vi "Calculate IV Average.vi"(8 "error in (no error)":errorcluster, 9 "Time Offset, s (0)":dbl format="%#_6p", 10 "Supply Line Handle in":refnum<k15>, 11 "Supply Line Measurements Results in":T1 {"Power (W)" format="%#_6p"; "Current (A)" format="%#_6p"; "Voltage (V)" format="%#_6p"}) -> (0 "error out":errorcluster, 3 "Supply Line Measurements Results out":T1 {"Power (W)" format="%#_6p"; "Current (A)" format="%#_6p"; "Voltage (V)" format="%#_6p"})   [LabVIEW 2016, in "RDLUtilities.lvlib"]
uses:
  RDLUtilities.lvlib
  Supply/Typedefs/Measurement Results.ctl
  <vilib>/Analysis/baseanly.llb/Mean (DBL).vi
  <vilib>/Analysis/NI_AALBase.lvlib
  Supply/Supply.lvlib
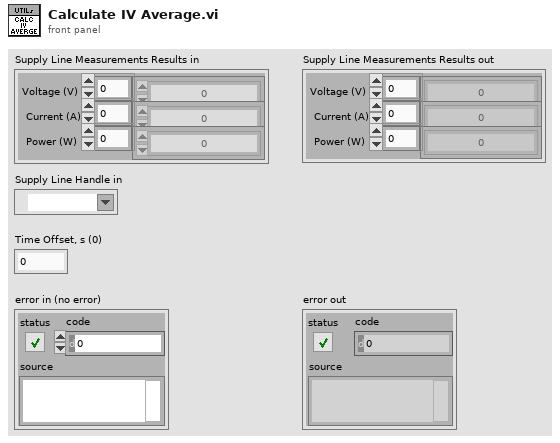
[diagram p1: front panel]
types:
  T1 = typedef "Supply.lvlib/Measurement Results.ctl" = cluster{"Voltage (V)":dbl[], "Current (A)":dbl[], "Power (W)":dbl[]}
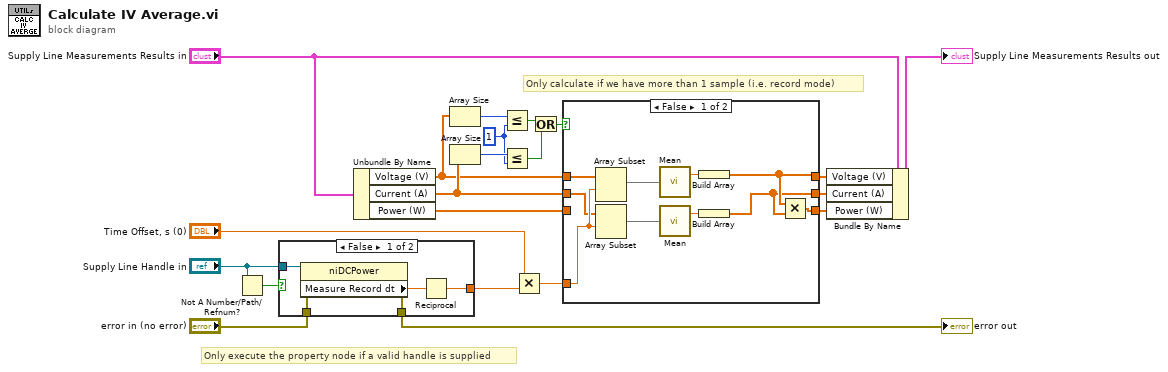
[diagram p0: block diagram]
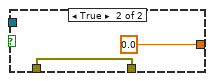
[diagram p3: hidden frame]
diagram:
  w5 = 1 ("y")
  # "Only calculate if we have more than 1 sample (i.e. record mode)"
  # "Only execute the property node if a valid handle is supplied"
  n1 = Not A Number/Path/Refnum?(number/path/refnum="Supply Line Handle in") -> (NaN/Path/Refnum?=w10:bool)
  n2 = case shown="False" w10 {
    tunnel: "error in (no error)" -> [w26 w28]
    tunnel: [w25 w28] -> w20
    tunnel: [w22 0.0 ("Measure Record dt")] -> w19
    tunnel: "Supply Line Handle in" -> [w23 _]
    frame False {
      n3 = property class="niDCPower"(reference=w23, error in=w26) -> (error out=w25:errorcluster, "Measure Record dt"=w24:dbl)  [unwired: 1 out]
      n4 = Reciprocal(x=w24) -> (1/x=w22:dbl)
    }
    frame True {
    }
  }
  "error out" <- w20
  n5 = Unbundle By Name("Supply Line Measurements Results in") -> ("Voltage (V)"=w8:dbl[], "Current (A)"=w9:dbl[], "Power (W)"=w1:dbl[])
  n6 = Array Size(array=w8) -> (size(s)=w7:i32)
  n7 = Array Size(array=w9) -> (size(s)=w6:i32)
  n8 = Less Or Equal?(x=w7, y=w5) -> (x <= y?=w4:bool)
  n9 = Less Or Equal?(x=w6, y=w5) -> (x <= y?=w3:bool)
  n10 = Multiply(x="Time Offset, s (0)", y=w19) -> (x*y=w17:dbl)
  n11 = Or(x=w4, y=w3) -> (x .or. y?=w2:bool)
  n12 = case shown="False" w2 {
    tunnel: w17 -> [w38 _]
    tunnel: [w33 w41] -> w14
    tunnel: [w32 w40] -> w13
    tunnel: [w31 w39] -> w12
    tunnel: w9 -> [w30 w40]
    tunnel: w8 -> [w29 w41]
    tunnel: w1 -> [_ w39]
    frame False {
      n13 = Array Subset(array=w29, index=w38) -> (w37:dbl[])  [unwired: 1 in]
      n14 = Array Subset(array=w30, index=w38) -> (w36:dbl[])  [unwired: 1 in]
      n15 = call-poly <vilib>:"Mean.vi"("X"=w37) -> ("mean"=w35:dbl)  [unwired: 1 out]
      n16 = call-poly <vilib>:"Mean.vi"("X"=w36) -> ("mean"=w34:dbl)  [unwired: 1 out]
      n17 = Build Array(w35) -> (w33:dbl[])
      n18 = Build Array(w34) -> (w32:dbl[])
      n19 = Multiply(x=w33, y=w32) -> (x*y=w31:dbl[])
    }
    frame True {
    }
  }
  n20 = Bundle By Name(cluster="Supply Line Measurements Results in", "Voltage (V)"=w14, "Current (A)"=w13, "Power (W)"=w12) -> (→"Supply Line Measurements Results out":T1)
